vi "Setup_PanelValueInit.vi"(8 "error in (no error)":errorcluster, 11 "Test.Maui 2.0.Panels in":refnum<class "Test.Maui 2.0.Panels.lvclass">) -> (0 "error out":errorcluster, 3 "Test.Maui 2.0.Panels out":refnum<class "Test.Maui 2.0.Panels.lvclass">)   [LabVIEW 2020, in "Test.Maui 2.0.Panels.lvclass"]
uses:
  Test.Maui 2.0.Panels.lvclass
  Maui 2.0/Maui 2.0.lvclass
  C:/Program Files (x86)/National Instruments/LabVIEW 2020/vi.lib/JKI/JKI SMO/SMO/SMO.lvclass
  Helper/Test Helper 1/Test Helper 1.lvclass
  Helper/Test Helper 2/Test Helper 2.lvclass
  C:/Users/Albro/Documents/GitHub/MAUI-Engine/lvsrc/Maui 2.0/Tests/Helper/Test Helper 1/Test Helper 1.lvclass
  Helper/Test Helper 3/Test Helper 3.lvclass
  Test.Maui 2.0.Panels.lvclass/Test.Maui 2.0.Panels.ctl
  <vilib>/JKI/JKI SMO/SMO/SMO.lvclass
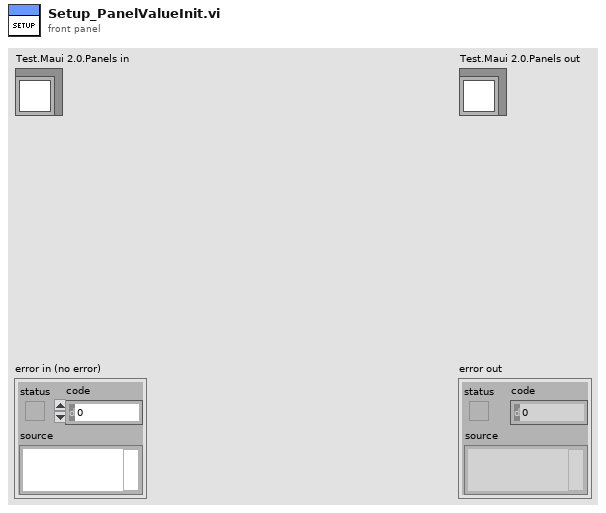
[diagram p1: front panel]
types:
  T1 = cluster{"Stop":refnum<user-event>, "Controls":refnum<user-event>}
  T2 = cluster{"Ring 2":refnum<vi>, "Sub Panel 2":refnum<vi>}[]
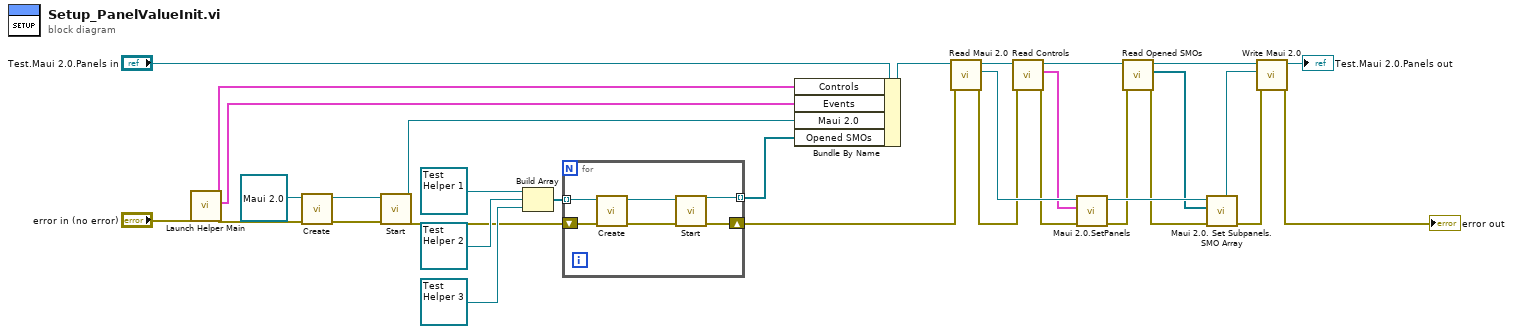
[diagram p0: block diagram]
diagram:
  n1 = call "Launch Helper Main.vi"("error in"="error in (no error)") -> ("error out"=w3:errorcluster, "Events"=w2:T1, "Controls"=w30:T2)  [unwired: 8 in]
  n2 = call <vilib>:"Create.vi"("error in (no error)"=w3, "SMO"=refnum<class "Maui 2.0.lvclass"> refnum ("Maui 2.0.lvclass")) -> ("error out"=w28:errorcluster, "SMO out"=w27:refnum<class "Maui 2.0.lvclass">)  [unwired: 7 in, 1 out]
  n3 = call <vilib>:"Start.vi"("error in (no error)"=w28, "SMO"=w27) -> ("error out"=w4:errorcluster, "SMO out"=w26:refnum<class "Maui 2.0.lvclass">)  [unwired: 8 in]
  n4 = Build Array(refnum<class "Test Helper 1.lvclass"> refnum ("Test Helper 1.lvclass"), refnum<class "Test Helper 2.lvclass"> refnum ("Test Helper 2.lvclass"), refnum<class "Test Helper 3.lvclass"> refnum ("Test Helper 3.lvclass")) -> (w22:refnum<class "Test Helper 1.lvclass">[])
  n5 = for {
    tunnel: w22 -> [w36] mode=indexing
    shift-right: [w34] -> w1
    shift-left: w4 -> [w35]
    tunnel: [w33] -> w21 mode=indexing
    n6 = call <vilib>:"Create.vi"("error in (no error)"=w35, "SMO"=w36) -> ("error out"=w37:errorcluster, "SMO out"=w38:refnum<class "Test Helper 1.lvclass">)  [unwired: 7 in, 1 out]
    n7 = call <vilib>:"Start.vi"("error in (no error)"=w37, "SMO"=w38) -> ("error out"=w34:errorcluster, "SMO out"=w33:refnum<class "Test Helper 1.lvclass">)  [unwired: 8 in]
  }
  n8 = Bundle By Name(cluster="Test.Maui 2.0.Panels in", "Controls"=w30, "Events"=w2, "Maui 2.0"=w26, "Opened SMOs"=w21) -> (w10:refnum<class "Test.Maui 2.0.Panels.lvclass">)
  n9 = call "Read Maui 2.0.vi"("error in (no error)"=w1, "Test.Maui 2.0.Panels in"=w10) -> ("error out"=w12:errorcluster, "Maui 2.0.lvclass"=w18:refnum<class "Maui 2.0.lvclass">, "Test.Maui 2.0.Panels out"=w19:refnum<class "Test.Maui 2.0.Panels.lvclass">)  [unwired: 7 in]
  n10 = call "Read Controls.vi"("error in (no error)"=w12, "Test.Maui 2.0.Panels in"=w19) -> ("error out"=w11:errorcluster, "Controls"=w17:T2, "Test.Maui 2.0.Panels out"=w16:refnum<class "Test.Maui 2.0.Panels.lvclass">)  [unwired: 7 in]
  n11 = call "Maui 2.0.SetPanels.vi"("error in (no error)"=w11, "Set Panels"=w17, "Maui 2.0"=w18) -> ("error out"=w14:errorcluster, "Maui 2.0 out"=w20:refnum<class "Maui 2.0.lvclass">)  [unwired: 7 in]
  n12 = call "Read Opened SMOs.vi"("error in (no error)"=w14, "Test.Maui 2.0.Panels in"=w16) -> ("error out"=w13:errorcluster, "Opened SMOs"=w15:refnum<class "Test Helper 1.lvclass">[], "Test.Maui 2.0.Panels out"=w9:refnum<class "Test.Maui 2.0.Panels.lvclass">)  [unwired: 7 in]
  n13 = call-dynamic "Maui 2.0. Set Subpanels.SMO Array.vi"("error in (no error)"=w13, "Subpanels in"=w15, "Maui 2.0 in"=w20) -> ("error out"=w6:errorcluster, "Maui 2.0 out"=w7:refnum<class "Maui 2.0.lvclass">)  [unwired: 6 in, 1 out]
  n14 = call "Write Maui 2.0.vi"("error in (no error)"=w6, "Maui 2.0.lvclass"=w7, "Test.Maui 2.0.Panels in"=w9) -> ("error out"=→"error out":errorcluster, "Test.Maui 2.0.Panels out"=→"Test.Maui 2.0.Panels out":refnum<class "Test.Maui 2.0.Panels.lvclass">)  [unwired: 7 in]
